vi "Get Identifier.vi"(8 "error in (no error)":errorcluster, 11 "Execution Unit in":refnum<class "Execution Unit.lvclass">) -> (0 "error out":errorcluster, 2 "Identifier":string, 3 "Execution Unit out":refnum<class "Execution Unit.lvclass">)   [LabVIEW 2020, in "Communication Bus Template Engine.lvlib" / "Interface.lvlib" / "Execution Unit.lvclass"]
uses:
  Execution Unit.lvclass
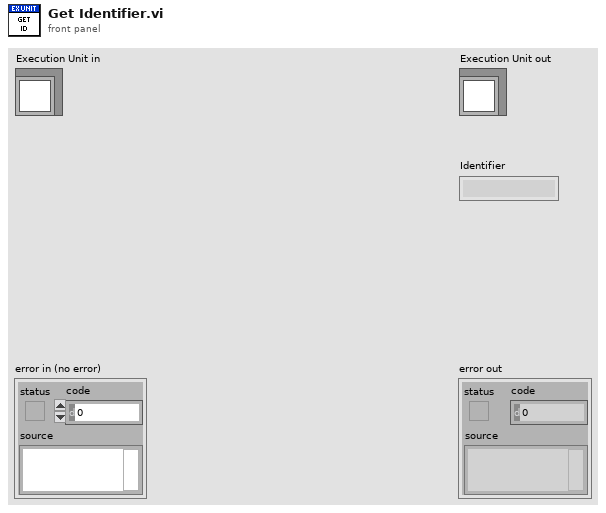
[diagram p1: front panel]
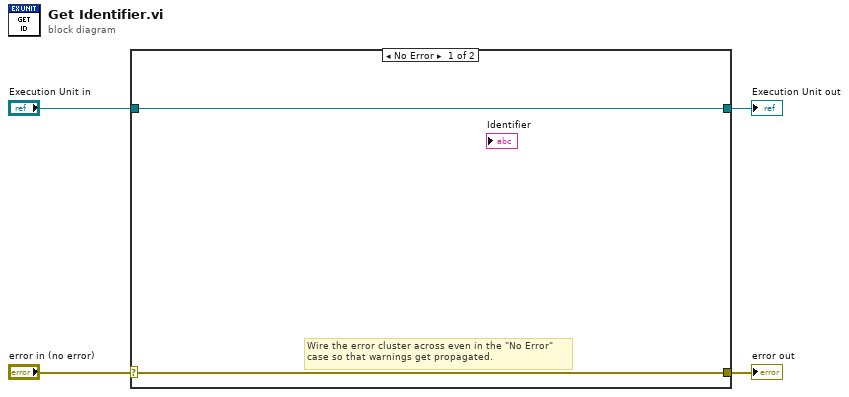
[diagram p0: block diagram]
diagram:
  n1 = case shown="No Error" "error in (no error)" {
    selector: "error in (no error)" -> [w5 w8]
    tunnel: [w5 w8] -> w3
    tunnel: [w6 w7] -> w1
    tunnel: "Execution Unit in" -> [w6 w7]
    frame No Error {
      # "Wire the error cluster across even in the \"No Error\"\ncase so that warnings get propagated."
    }
    frame Error {
    }
  }
  "error out" <- w3
  "Execution Unit out" <- w1
